vi "Length_2.vi"() -> ()   [LabVIEW 2020]
uses:
  Support/Controls/Cmd_Mouse Popup.ctl
  Support/Controls/Clst_Initialize Input.ctl
  Support/Controls/Clst_Result inspec.ctl
  Support/Controls/Cmd_Var Data IO.ctl
  Variables/Global_Cal Info.vi
panel:
  in  "불리언 2":bool=TRUE caption="평행도"
  in  "불리언 1":bool=TRUE caption="평면도"
  in  "Measured 3":string[][](table) caption="평행도"
  out "STD set":string[][](table) caption="○ 기준기 조합 (값)"
  in  "Measured 2":string[][](table) caption="평면도"
  in  "표시방식":string(combo)
  out "단위":string
  out "최대범위":string
  in  "Spec 변경":bool
  in  "Random":bool
  out "Resolution":string[][](table) caption="평면도"
  out "Spec":string[][](table) caption="평행도"
  out "제목":string
  out "에러 출력":errorcluster
  out "Condition":string[][](table) caption="2. 직선성 시험"
  in  "최소눈금":string(combo)
  in  "Measured":string[][](table) caption="평면도"
  out "Load?":bool
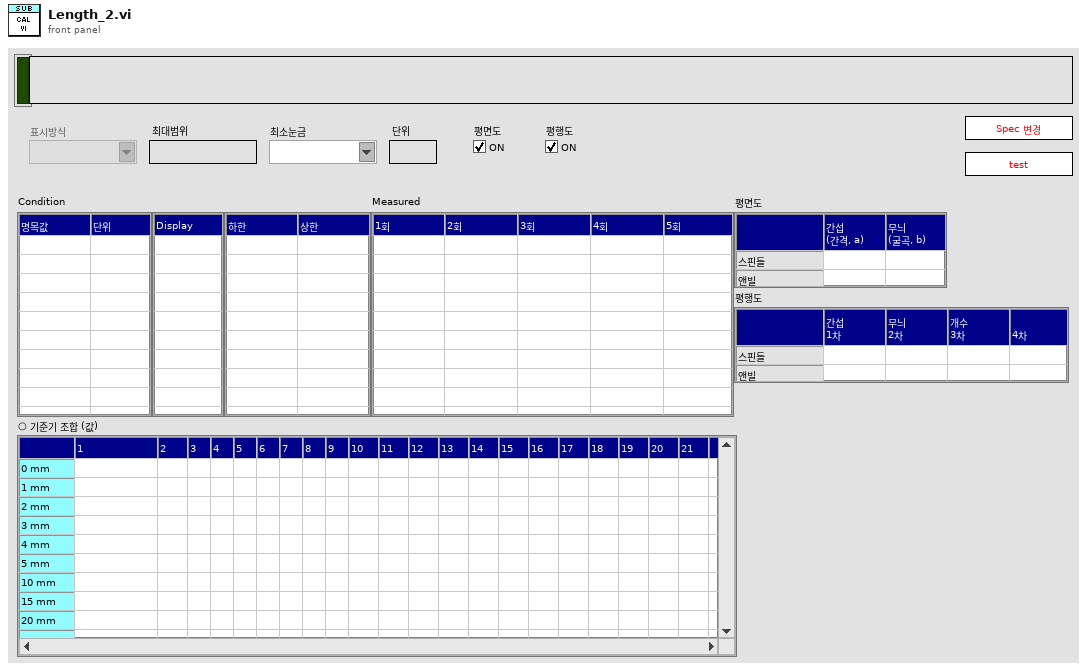
[diagram p1: front panel]
types:
  T1 = typedef "Cmd_Mouse Popup.ctl" = enum16{"활성화", "메뉴선택"}
  T2 = cluster{"Shift":bool, "Ctrl":bool, "Alt":bool, "Cmd":bool, "Opt":bool}
  T3 = typedef "Clst_Initialize Input.ctl" = cluster{"Initialize 1":cluster{"Condition":refnum<vi>[], "Spec":refnum<vi>[], "Measured":refnum<vi>[], "Resolution":refnum<vi>[], "Func_ext":string, "제목":refnum<vi>, "Measured_ADJ":refnum<vi>[]}, "Initialize 2":cluster{"문자열":refnum<vi>[], "콤보박스":refnum<vi>[], "링":refnum<vi>[], "열거형":refnum<vi>[], "테이블":refnum<vi>[], "여러열":refnum<vi>[], "디지털(DBL)":refnum<vi>[], "3D string":refnum<vi>[], "ctrl":refnum<vi>[], "boolean":refnum<vi>[]}}
  T4 = typedef "Clst_Result inspec.ctl" = cluster{"분해능":string, "문자열 1":string, "문자열 2":string, "숫자형 1":i32, "숫자형 2":i32, "숫자형 3":dbl, "문자배열 1D":string[], "문자배열 2D":string[][], "문자배열 3D":string[][][], "문자배열 4D":string[][][][], "불리언 1D":bool[]}
  T5 = typedef "Cmd_Var Data IO.ctl" = enum16{"Condition", "Condition Default", "Condition_Temp", "Resolution", "Resolution Default", "Resolution Old", "Spec", "Spec Default", "Spec Old", "Spec Temp", "Result", "Result2", "Result3", "Result_Temp", "Result_ADJ", "Result_ADJ2", "STD1", "STD2", "STD3", "STD4", "STD5", "STD Temp", "CMC", "CMC Default"}
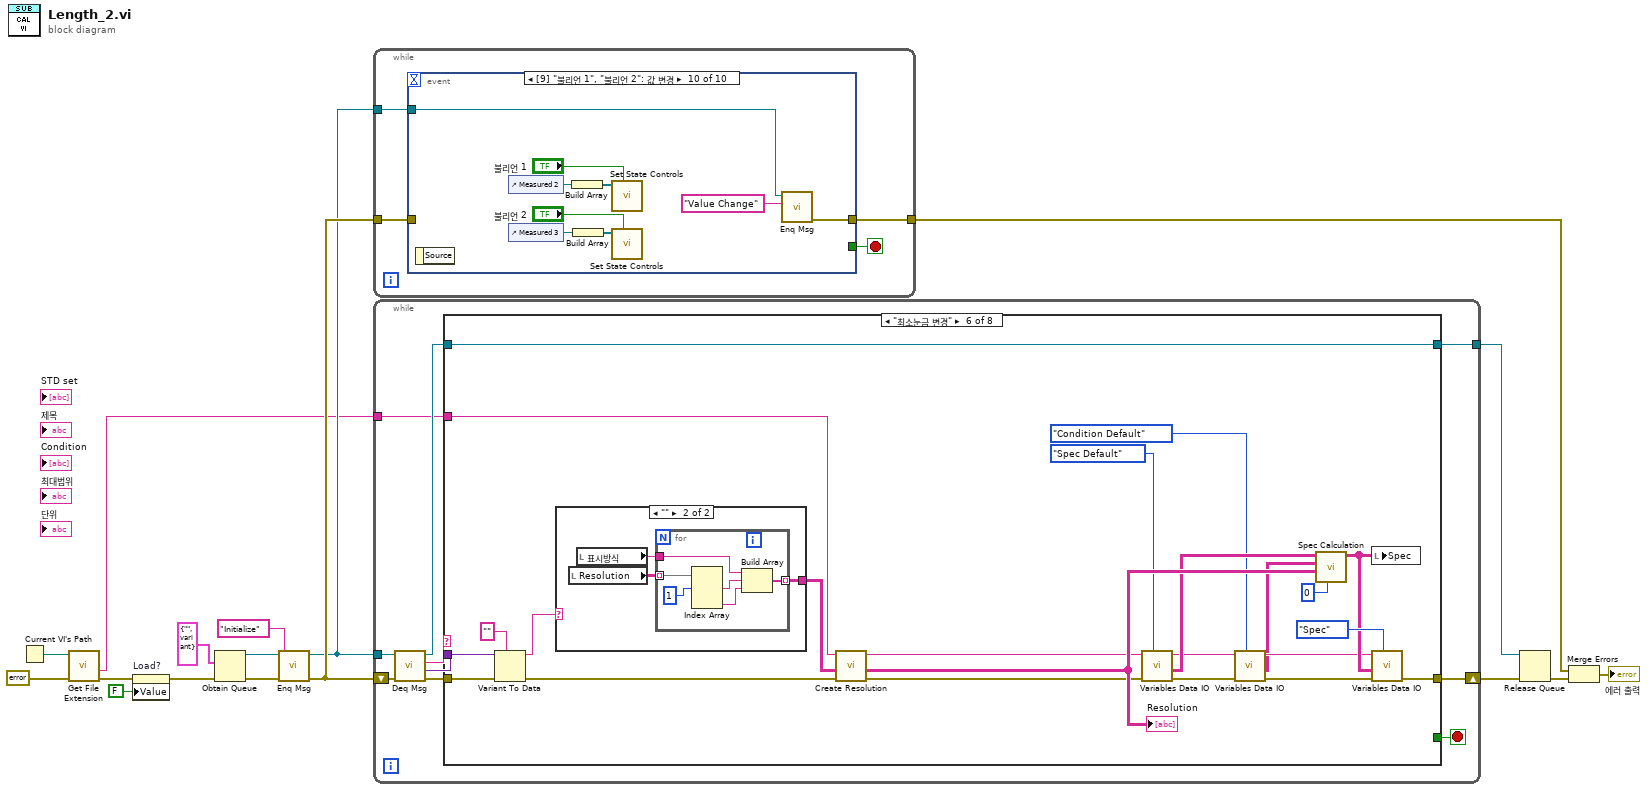
[diagram p0: block diagram]
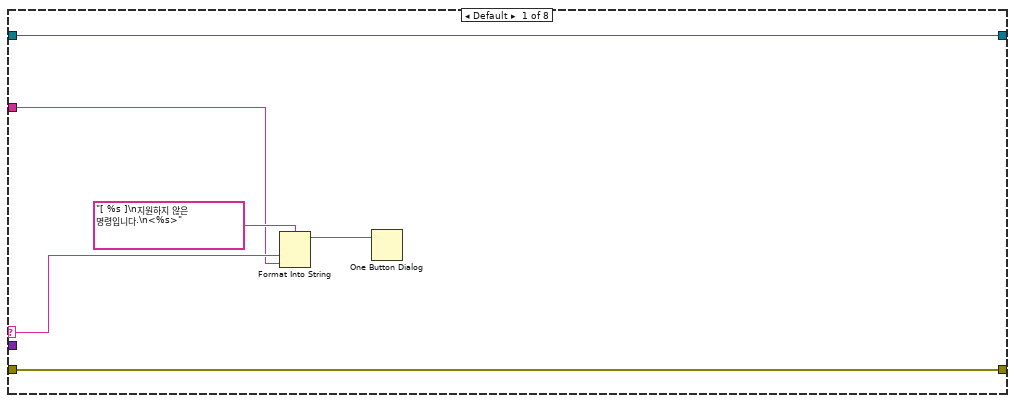
[diagram p2: hidden frame]
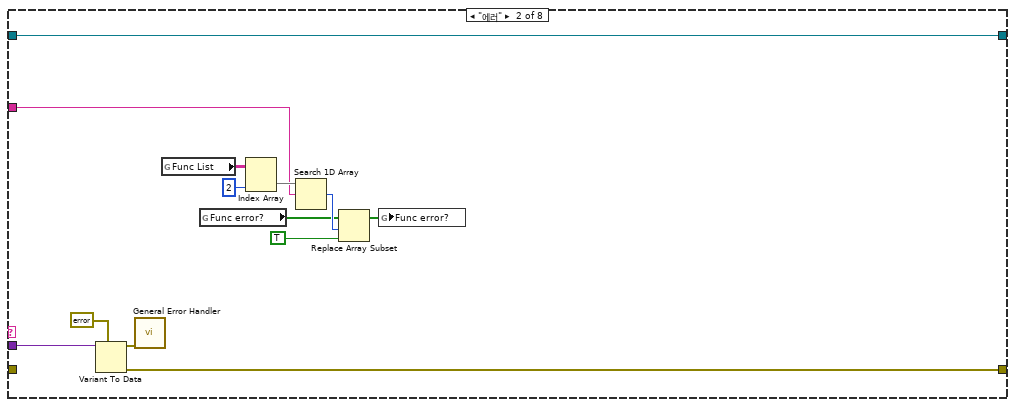
[diagram p3: hidden frame]
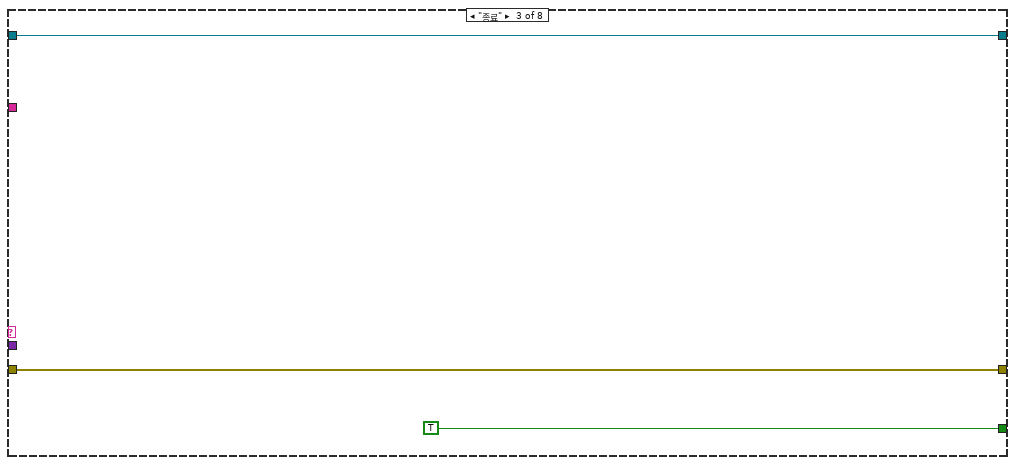
[diagram p4: hidden frame]
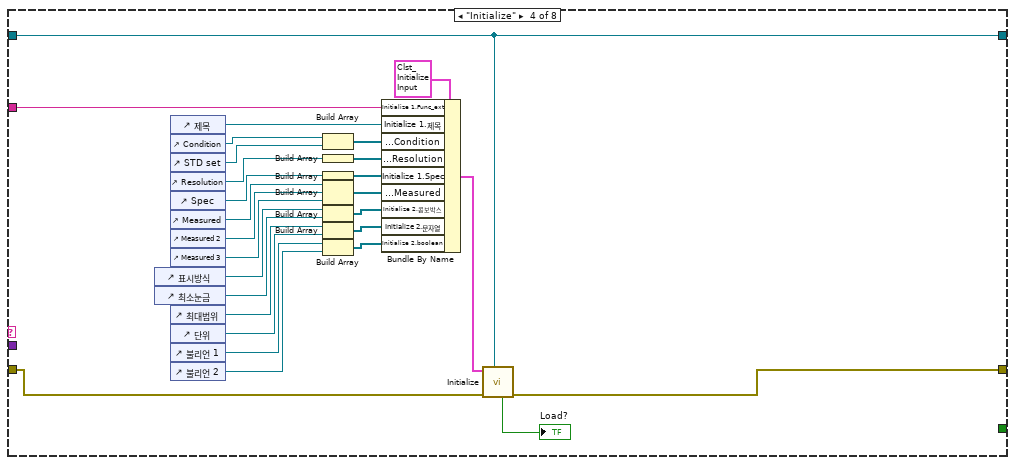
[diagram p5: hidden frame]
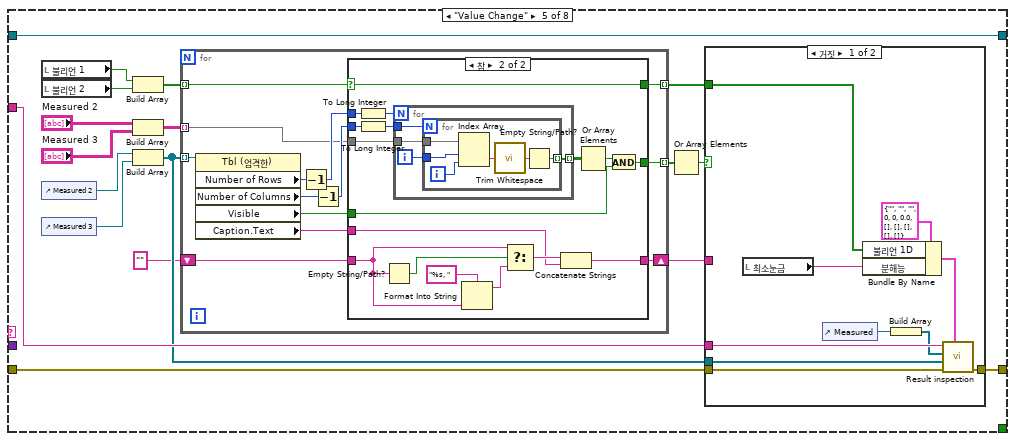
[diagram p6: hidden frame]
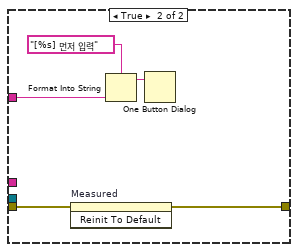
[diagram p8: hidden frame]
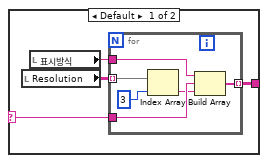
[diagram p9: hidden frame]
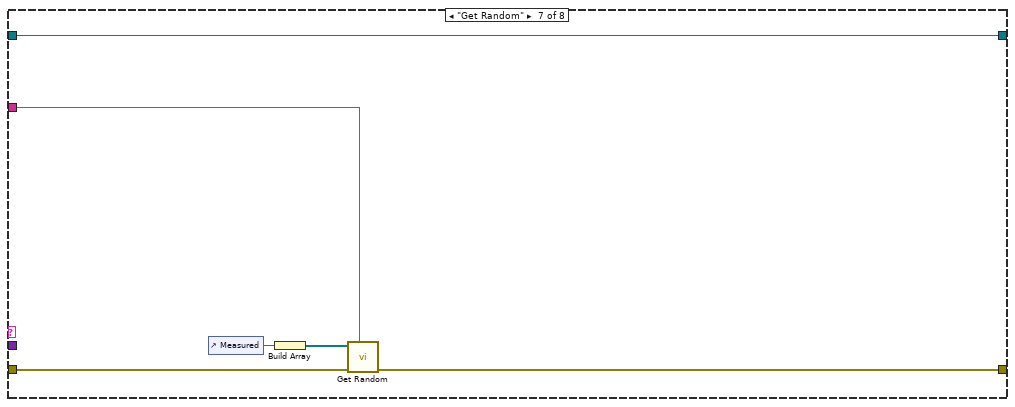
[diagram p10: hidden frame]
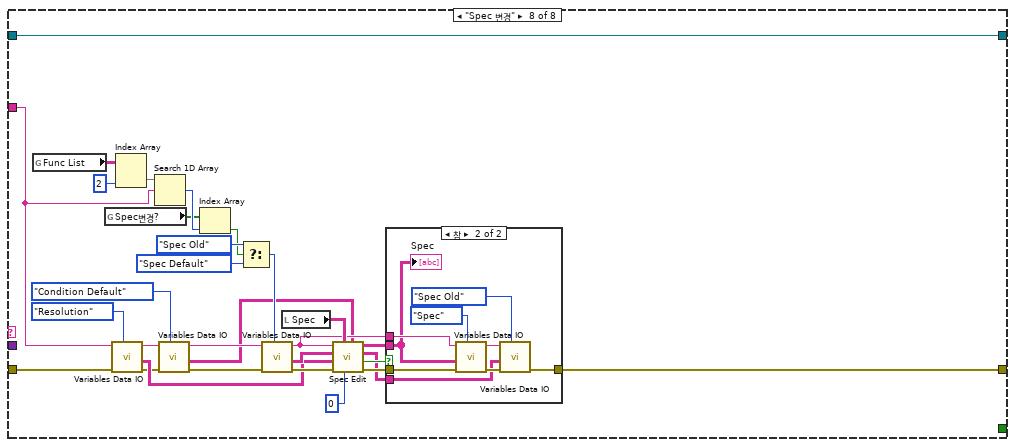
[diagram p11: hidden frame]
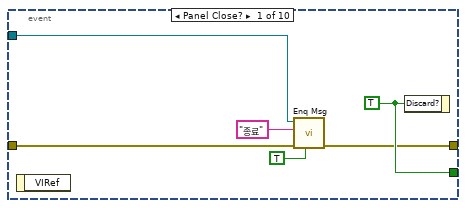
[diagram p13: hidden frame]
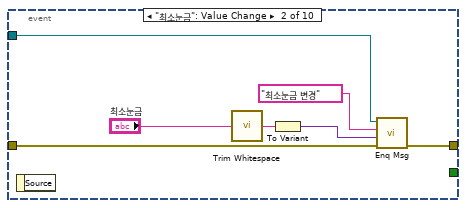
[diagram p14: hidden frame]
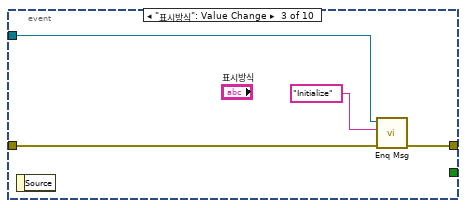
[diagram p15: hidden frame]
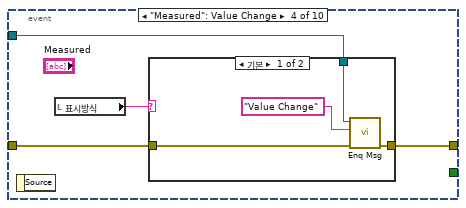
[diagram p16: hidden frame]
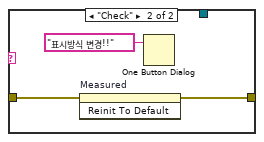
[diagram p17: hidden frame]
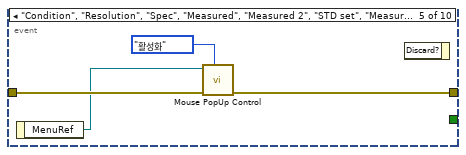
[diagram p18: hidden frame]
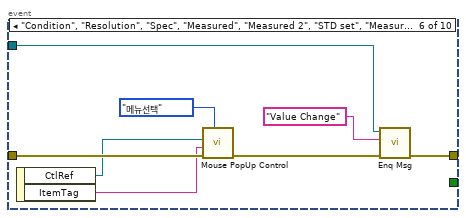
[diagram p19: hidden frame]
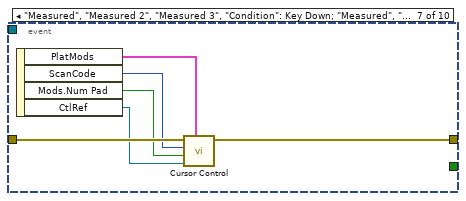
[diagram p20: hidden frame]
diagram:
  n1 = Current VI's Path() -> (path=w5:path)
  n2 = call <vilib>:"Get File Extension.vi"("error in (no error)"=errorcluster {"status"=FALSE, "code"=0, "source"=""} ("에러 상수"), "file"=w5) -> ("error out"=w3:errorcluster, "filename without extension"=w4:string)  [unwired: 5 in, 3 out]
  n3 = property on="Load?" class="Bool (엄격한)"(error in=w3, "Value"=FALSE ("Load?")) -> (error out=w2:errorcluster)  [unwired: 1 in, 1 out]
  n4 = Obtain Queue(element data type=cluster{"메세지":string, "값":variant} {"메세지"="", "값"=variant} ("Message Cluster"), error in (no error)=w2) -> (queue out=w14:refnum<queue>, error out=w16:errorcluster)  [unwired: 3 in, 1 out]
  n5 = call "Enq Msg.vi"("에러 입력(에러 없음)"=w16, "메세지"="Initialize", "큐 입력"=w14) -> ("에러 출력"=w15:errorcluster, "큐 출력"=w12:refnum<queue>)  [unwired: 7 in]
  n6 = while {
    tunnel: w15 -> [w19]
    tunnel: w12 -> [w20]
    tunnel: [w18] -> w9
    stop <- w21 stop-if-true
    n7 = event shown="[9] \"불리언 1\", \"불리언 2\": 값 변경" {
      selector: _ -> [_ _ _ _ _ _ _ _ _ _]
      dyn-events: _ -> [_ _ _ _ _ _ _ _ _ _]
      timeout: _ -> [_ _ _ _ _ _ _ _ _ _]
      tunnel: [w27 _ _ _ _ _ _ _ _ _] -> w21
      tunnel: w20 -> [w25 w33 w37 w42 _ w54 _ w72 w76 w79]
      tunnel: w19 -> [w26 w34 w38 w40 w53 w61 w67 w73 w77 _]
      tunnel: [w23 w32 w36 w41 w52 w55 w66 w68 w75 w80] -> w18
      event Panel Close? {
        w27 = TRUE ("버림?")
        n8 = event-data() -> ()  [unwired: 1 in, 1 out]
        n9 = call "Enq Msg.vi"("우선순위 메시지?"=TRUE, "에러 입력(에러 없음)"=w26, "메세지"="종료", "큐 입력"=w25) -> ("에러 출력"=w23:errorcluster)  [unwired: 6 in, 1 out]
        n10 = event-data("Discard?"=w27) -> ()  [unwired: 1 in, 1 out]
      }
      event "최소눈금": Value Change {
        n11 = event-data() -> ()  [unwired: 1 in, 1 out]
        n12 = call <vilib>:"Trim Whitespace.vi"("string"="최소눈금") -> ("trimmed string"=w30:string)  [unwired: 1 in]
        n13 = To Variant(anything=w30) -> (Variant=w28:variant)
        n14 = call "Enq Msg.vi"("에러 입력(에러 없음)"=w34, "값"=w28, "메세지"="최소눈금 변경", "큐 입력"=w33) -> ("에러 출력"=w32:errorcluster)  [unwired: 6 in, 1 out]
      }
      event "표시방식": Value Change {
        n15 = event-data() -> ()  [unwired: 1 in, 1 out]
        n16 = call "Enq Msg.vi"("에러 입력(에러 없음)"=w38, "메세지"="Initialize", "큐 입력"=w37) -> ("에러 출력"=w36:errorcluster)  [unwired: 7 in, 1 out]
      }
      event "Measured": Value Change {
        n17 = event-data() -> ()  [unwired: 1 in, 1 out]
        n18 = local read "표시방식"() -> (w39:string)
        n19 = case shown="기본" w39 {
          tunnel: w42 -> [w46 _]
          tunnel: [w45 w47] -> w41
          tunnel: w40 -> [w44 w48]
          frame Default {
            n20 = call "Enq Msg.vi"("에러 입력(에러 없음)"=w44, "메세지"="Value Change", "큐 입력"=w46) -> ("에러 출력"=w45:errorcluster)  [unwired: 7 in, 1 out]
          }
          frame "Check" {
            n21 = invoke on="Measured" class="Tbl (엄격한)" method="Reinit To Default"(error in=w48) -> (error out=w47:errorcluster)  [unwired: 2 in, 2 out]
            n22 = One Button Dialog(message="표시방식 변경!!" ("메시지")) -> ()  [unwired: 1 in, 1 out]
          }
        }
      }
      event "Condition", "Resolution", "Spec", "Measured", "Measured 2", "STD set", "Measured 3": Shortcut Menu Activation? {
        n23 = event-data() -> ("MenuRef"=w51:refnum<k9>)  [unwired: 1 in]
        n24 = call "Mouse PopUp Control.vi"("type"=Cmd_Mouse_Popup."활성화", "error in"=w53, "메뉴 참조"=w51) -> ("error out"=w52:errorcluster)  [unwired: 8 in]
        n25 = event-data() -> ()  [unwired: 2 in, 1 out]
      }
      event "Condition", "Resolution", "Spec", "Measured", "Measured 2", "STD set", "Measured 3": Shortcut Menu Selection (User) {
        n26 = event-data() -> ("CtlRef"=w59:refnum<vi>, "ItemTag"=w58:string)  [unwired: 1 in]
        n27 = call "Mouse PopUp Control.vi"("type"=Cmd_Mouse_Popup."메뉴선택", "error in"=w61, "아이템 태그"=w58, "Tbl 참조 번호"=w59) -> ("error out"=w56:errorcluster)  [unwired: 7 in]
        n28 = call "Enq Msg.vi"("에러 입력(에러 없음)"=w56, "메세지"="Value Change", "큐 입력"=w54) -> ("에러 출력"=w55:errorcluster)  [unwired: 7 in, 1 out]
      }
      event "Measured", "Measured 2", "Measured 3", "Condition": Key Down; "Measured", "Measured 2", "Measured 3", "Condition": Key Repeat {
        n29 = event-data() -> ("PlatMods"=w62:T2, "ScanCode"=w65:i16, "Mods.Num Pad"=w64:bool, "CtlRef"=w63:refnum<vi>)  [unwired: 1 in]
        n30 = call "Cursor Control.vi"("플랫폼 조합키"=w62, "참조"=w63, "Num Pad"=w64, "ScanCode"=w65, "error in"=w67) -> ("error out"=w66:errorcluster)  [unwired: 5 in, 1 out]
      }
      event "Random": Value Change {
        n31 = event-data() -> ()  [unwired: 1 in, 1 out]
        n32 = call "Enq Msg.vi"("에러 입력(에러 없음)"=w73, "메세지"="Get Random", "큐 입력"=w72) -> ("에러 출력"=w71:errorcluster, "큐 출력"=w70:refnum<queue>)  [unwired: 7 in]
        n33 = call "Enq Msg.vi"("에러 입력(에러 없음)"=w71, "메세지"="Value Change", "큐 입력"=w70) -> ("에러 출력"=w68:errorcluster)  [unwired: 7 in, 1 out]
      }
      event "Spec 변경": Value Change {
        n34 = event-data() -> ()  [unwired: 1 in, 1 out]
        n35 = call "Enq Msg.vi"("에러 입력(에러 없음)"=w77, "메세지"="Spec 변경", "큐 입력"=w76) -> ("에러 출력"=w75:errorcluster)  [unwired: 7 in, 1 out]
      }
      event "불리언 1", "불리언 2": Value Change {
        n36 = event-data() -> ()  [unwired: 1 in, 1 out]
        n37 = control-ref of="Measured 2"() -> (w87:refnum<vi>)
        n38 = control-ref of="Measured 3"() -> (w83:refnum<vi>)
        n39 = Build Array(w87) -> (w86:refnum<vi>[])
        n40 = Build Array(w83) -> (w84:refnum<vi>[])
        n41 = call "Set State Controls.vi"("활성화 (F)"="불리언 1", "컨트롤 참조 배열 in"=w86) -> ()  [unwired: 8 in, 2 out]
        n42 = call "Set State Controls.vi"("활성화 (F)"="불리언 2", "컨트롤 참조 배열 in"=w84) -> ()  [unwired: 8 in, 2 out]
        n43 = call "Enq Msg.vi"("메세지"="Value Change", "큐 입력"=w79) -> ("에러 출력"=w80:errorcluster)  [unwired: 8 in, 1 out]
      }
    }
  }
  n44 = while {
    shift-right: [w97] -> w11
    shift-left: w15 -> [w96]
    tunnel: w12 -> [w94]
    tunnel: [w89] -> w10
    tunnel: w4 -> [w88]
    stop <- w90 stop-if-true
    n45 = call "Deq Msg.vi"("에러 입력(에러 없음)"=w96, "큐 입력"=w94) -> ("에러 출력"=w95:errorcluster, "값"=w91:variant, "메세지"=w93:string, "큐 출력"=w92:refnum<queue>)  [unwired: 6 in]
    n46 = case shown="\"최소눈금 변경\"" w93 {
      selector: w93 -> [w99 _ _ _ _ _ _ _]
      tunnel: w95 -> [w103 _ w119 w147 w151 w243 w265 w292]
      tunnel: [w103 w113 w119 w137 w164 w236 w266 w295] -> w97
      tunnel: w92 -> [w102 w112 w117 w131 w165 w244 w269 w299]
      tunnel: w91 -> [_ w114 _ _ _ w242 _ _]
      tunnel: [_ _ TRUE ("버림?") _ _ _ _ _] -> w90
      tunnel: [w102 w112 w117 w131 w165 w244 w269 w299] -> w89
      tunnel: w88 -> [w98 w104 _ w132 w163 w240 w264 w277]
      frame Default {
        n47 = Format Into String(format string="[ %s ]\n지원하지 않은 명령입니다.\n<%s>" ("메시지"), w99, w98) -> (resulting string=w100:string)  [unwired: 2 in, 1 out]
        n48 = One Button Dialog(message=w100) -> ()  [unwired: 1 in, 1 out]
      }
      frame "에러" {
        n49 = Variant To Data(type=errorcluster {"status"=FALSE, "code"=0, "source"=""} ("에러 출력"), Variant=w114) -> (data=w116:errorcluster, error out=w113:errorcluster)  [unwired: 1 in]
        n50 = call <vilib>:"General Error Handler.vi"("error in (no error)"=w116) -> ()  [unwired: 10 in, 5 out]
        n51 = global read "Global_Cal Info.vi" "Func List"() -> (w106:string[][])
        n52 = global read "Global_Cal Info.vi" "Func error?"() -> (w109:bool[])
        n53 = Index Array(array=w106, index (col)=2 ("비활성화된 인덱스 (열)")) -> (element=w107:string[])  [unwired: 1 in]
        n54 = Search 1D Array(1D array=w107, element=w104) -> (index of element=w110:i32)  [unwired: 1 in]
        n55 = Replace Array Subset(array=w109, new element=TRUE ("새 원소/부분배열"), index=w110) -> (w111:bool[])
        n56 = global write "Global_Cal Info.vi" "Func error?"(w111) -> ()
      }
      frame "종료" {
      }
      frame "Initialize" {
        n57 = control-ref of="표시방식"() -> (w130:refnum<vi>)
        n58 = control-ref of="최소눈금"() -> (w140:refnum<vi>)
        n59 = control-ref of="제목"() -> (w138:refnum<vi>)
        n60 = control-ref of="Condition"() -> (w144:refnum<vi>)
        n61 = control-ref of="STD set"() -> (w125:refnum<vi>)
        n62 = control-ref of="Resolution"() -> (w133:refnum<vi>)
        n63 = control-ref of="Spec"() -> (w136:refnum<vi>)
        n64 = control-ref of="Measured"() -> (w141:refnum<vi>)
        n65 = control-ref of="Measured 2"() -> (w126:refnum<vi>)
        n66 = control-ref of="Measured 3"() -> (w124:refnum<vi>)
        n67 = control-ref of="최대범위"() -> (w127:refnum<vi>)
        n68 = control-ref of="단위"() -> (w129:refnum<vi>)
        n69 = control-ref of="불리언 1"() -> (w123:refnum<vi>)
        n70 = control-ref of="불리언 2"() -> (w122:refnum<vi>)
        n71 = Build Array(w144, w125) -> (w143:refnum<vi>[])
        n72 = Build Array(w133) -> (w134:refnum<vi>[])
        n73 = Build Array(w136) -> (w135:refnum<vi>[])
        n74 = Build Array(w141, w126, w124) -> (w142:refnum<vi>[])
        n75 = Build Array(w130, w140) -> (w139:refnum<vi>[])
        n76 = Build Array(w127, w129) -> (w128:refnum<vi>[])
        n77 = Build Array(w123, w122) -> (w121:refnum<vi>[])
        n78 = Bundle By Name(cluster=T3 {"Initialize 1"={"Condition"=[], "Spec"=[], "Measured"=[], "Resolution"=[], "Func_ext"="", "제목"=refnum, "Measured_ADJ"=[]}, "Initialize 2"={"문자열"=[], "콤보박스"=[], "링"=[], "열거형"=[], "테이블"=[], "여러열"=[], "디지털(DBL)"=[], "3D string"=[], "ctrl"=[], "boolean"=[]}} ("입력 클러스터"), "Initialize 1.Func_ext"=w132, "Initialize 1.제목"=w138, "Initialize 1.Condition"=w143, "Initialize 1.Resolution"=w134, "Initialize 1.Spec"=w135, "Initialize 1.Measured"=w142, "Initialize 2.콤보박스"=w139, "Initialize 2.문자열"=w128, "Initialize 2.boolean"=w121) -> (w145:T3)
        n79 = call "Initialize.vi"("큐 입력"=w131, "error in"=w147, "입력 클러스터"=w145) -> ("error out"=w137:errorcluster, "Load?"=→"Load?":bool)  [unwired: 5 in, 2 out]
      }
      frame "Value Change" {
        n80 = local read "불리언 1"() -> (w156:bool)
        n81 = local read "불리언 2"() -> (w157:bool)
        n82 = control-ref of="Measured 2"() -> (w154:refnum<vi>)
        n83 = control-ref of="Measured 3"() -> (w160:refnum<vi>)
        n84 = Build Array(w156, w157) -> (w158:bool[])
        n85 = Build Array("Measured 2", "Measured 3") -> (w155:string[][][])
        n86 = Build Array(w154, w160) -> (w152:refnum<vi>[])
        n87 = for {
          tunnel: w152 -> [w178] mode=indexing
          tunnel: w155 -> [w173] mode=indexing
          tunnel: w158 -> [w170] mode=indexing
          tunnel: [w169] -> w159 mode=indexing
          shift-right: [w167] -> w149
          shift-left: "" ("Caption.Text") -> [w168]
          tunnel: [w166] -> w148 mode=indexing
          n88 = property on="프로퍼티 노드" class="Tbl (엄격한)"(reference=w178) -> ("Number of Rows"=w177:u32, "Number of Columns"=w176:u32, "Visible"=w172:bool, "Caption.Text"=w171:string)  [unwired: 1 in, 2 out]
          n89 = Decrement(x=w177) -> (x-1=w175:u32)
          n90 = Decrement(x=w176) -> (x-1=w174:u32)
          n91 = case shown="참" w170 {
            selector: w170 -> [_ w180]
            tunnel: w173 -> [_ w192]
            tunnel: w175 -> [_ w196]
            tunnel: w172 -> [_ w189]
            tunnel: w174 -> [_ w195]
            tunnel: [_ w188] -> w169
            tunnel: w171 -> [_ w181]
            tunnel: w168 -> [w179 w183]
            tunnel: [w179 w182] -> w167
            tunnel: [_ w180] -> w166
            frame False {
            }
            frame True {
              n92 = To Long Integer(number=w196) -> (32bit integer=w194:i32)
              n93 = To Long Integer(number=w195) -> (32bit integer=w193:i32)
              n94 = Empty String/Path?(string/path=w183) -> (empty?=w187:bool)
              n95 = for {
                N: w194 -> [_]
                tunnel: w192 -> [w199]
                tunnel: w193 -> [w200]
                tunnel: [w198] -> w191 mode=indexing
                i -> [w197]
                n96 = for {
                  N: w200 -> [_]
                  tunnel: w199 -> [w204]
                  tunnel: [w205] -> w198 mode=indexing
                  tunnel: w197 -> [w202]
                  i -> [w201]
                  n97 = Index Array(array=w204, index (row)=w202, index (col)=w201) -> (element=w203:string)
                  n98 = call <vilib>:"Trim Whitespace.vi"("string"=w203) -> ("trimmed string"=w206:string)  [unwired: 1 in]
                  n99 = Empty String/Path?(string/path=w206) -> (empty?=w205:bool)
                }
              }
              n100 = Format Into String(format string="%s, " ("포맷 문자열"), w183) -> (resulting string=w185:string)  [unwired: 2 in, 1 out]
              n101 = Select(t=w183, s=w187, f=w185) -> (s? t:f=w184:string)
              n102 = Concatenate Strings(w184, w181) -> (w182:string)
              n103 = Or Array Elements(Boolean array=w191) -> (logical OR=w190:bool)
              n104 = And(x=w190, y=w189) -> (x .and. y?=w188:bool)
            }
          }
        }
        n105 = Or Array Elements(Boolean array=w159) -> (logical OR=w153:bool)
        n106 = case shown="거짓" w153 {
          tunnel: [w216 w219] -> w164
          tunnel: w163 -> [w215 _]
          tunnel: w152 -> [w209 _]
          tunnel: w151 -> [w208 w218]
          tunnel: w149 -> [_ w217]
          tunnel: w148 -> [w207 _]
          frame False {
            n107 = local read "최소눈금"() -> (w211:string)
            n108 = control-ref of="Measured"() -> (w214:refnum<vi>)
            n109 = Bundle By Name(cluster=T4 {"분해능"="", "문자열 1"="", "문자열 2"="", "숫자형 1"=0, "숫자형 2"=0, "숫자형 3"=0.0, "문자배열 1D"=[], "문자배열 2D"=[], "문자배열 3D"=[], "문자배열 4D"=[], "불리언 1D"=[]} ("입력 클러스터"), "불리언 1D"=w207, "분해능"=w211) -> (w210:T4)
            n110 = Build Array(w214) -> (w213:refnum<vi>[])
            n111 = call "Result inspection.vi"("입력 클러스터"=w210, "error in"=w208, "Ref. Data (excluded)"=w209, "Ref. Data (Inspection)"=w213, "Func ext"=w215) -> ("error out"=w216:errorcluster)  [unwired: 3 in, 3 out]
          }
          frame True {
            n112 = invoke on="Measured" class="Tbl (엄격한)" method="Reinit To Default"(error in=w218) -> (error out=w219:errorcluster)  [unwired: 2 in, 2 out]
            n113 = Format Into String(format string="[%s] 먼저 입력" ("포맷 문자열"), w217) -> (resulting string=w220:string)  [unwired: 2 in, 1 out]
            n114 = One Button Dialog(message=w220) -> ()  [unwired: 1 in, 1 out]
          }
        }
      }
      frame "최소눈금 변경" {
        n115 = Variant To Data(error in=w243, type="", Variant=w242) -> (data=w229:string, error out=w231:errorcluster)
        n116 = case shown="\"\"" w229 {
          selector: w229 -> [w245 _]
          tunnel: [w248 w257] -> w230
          frame Default {
            n117 = local read "Resolution"() -> (w247:string[][])
            n118 = local read "표시방식"() -> (w246:string)
            n119 = for {
              tunnel: w247 -> [w254] mode=indexing
              tunnel: w245 -> [w253]
              tunnel: [w251] -> w248 mode=indexing
              tunnel: w246 -> [w250]
              n120 = Index Array(array=w254, index=3 ("인덱스")) -> (element=w252:string)
              n121 = Build Array(w250, w253, w252) -> (w251:string[])
            }
          }
          frame "" {
            n122 = local read "Resolution"() -> (w256:string[][])
            n123 = local read "표시방식"() -> (w255:string)
            n124 = for {
              tunnel: w256 -> [w263] mode=indexing
              tunnel: [w262] -> w257 mode=indexing
              tunnel: w255 -> [w261]
              n125 = Index Array(array=w263, index #1=1 ("인덱스")) -> (element #1=w259:string, element #3=w258:string)  [unwired: 2 in, 1 out]
              n126 = Build Array(w261, w259, w258) -> (w262:string[])
            }
          }
        }
        n127 = call "Create Resolution.vi"("에러 입력(에러 없음)"=w231, "Resolution"=w230, "Func_ext"=w240) -> ("에러 출력"=w234:errorcluster, "Resolution Out"=w237:string[][], "Func_ext 출력"=w233:string)  [unwired: 6 in]
        "Resolution" <- w237
        n128 = call "Variables Data IO.vi"("Select"=Cmd_Var_Data_IO."Spec Default", "error in"=w234, "Func_ext"=w233) -> ("error out"=w225:errorcluster, "Data Out"=w232:string[][], "Func_ext Out"=w226:string)  [unwired: 6 in]
        n129 = call "Variables Data IO.vi"("Select"=Cmd_Var_Data_IO."Condition Default", "error in"=w225, "Func_ext"=w226) -> ("error out"=w223:errorcluster, "Data Out"=w222:string[][], "Func_ext Out"=w224:string)  [unwired: 6 in]
        n130 = call "Spec Calculation.vi"("기준값 열번호"=0 ("열번호(기준값)"), "Resolution"=w237, "Condition in"=w222, "Spec Default"=w232) -> ("Spec out"=w228:string[][])  [unwired: 6 in, 1 out]
        n131 = local write "Spec"(w228) -> ()
        n132 = call "Variables Data IO.vi"("Select"=Cmd_Var_Data_IO."Spec", "error in"=w223, "Data In"=w228, "Func_ext"=w224) -> ("error out"=w236:errorcluster)  [unwired: 5 in, 2 out]
      }
      frame "Get Random" {
        n133 = control-ref of="Measured"() -> (w268:refnum<vi>)
        n134 = Build Array(w268) -> (w267:refnum<vi>[])
        n135 = call "Get Random.vi"("Func_Ext"=w264, "에러 입력"=w265, "Meas"=w267) -> ("에러 출력"=w266:errorcluster)  [unwired: 7 in, 1 out]
      }
      frame "Spec 변경" {
        n136 = global read "Global_Cal Info.vi" "Func List"() -> (w282:string[][])
        n137 = global read "Global_Cal Info.vi" "Spec변경?"() -> (w278:bool[])
        n138 = call "Variables Data IO.vi"("Select"=Cmd_Var_Data_IO."Resolution", "error in"=w292, "Func_ext"=w277) -> ("error out"=w275:errorcluster, "Data Out"=w286:string[][], "Func_ext Out"=w273:string)  [unwired: 6 in]
        n139 = Index Array(array=w282, index (col)=2 ("비활성화된 인덱스 (열)")) -> (element=w280:string[])  [unwired: 1 in]
        n140 = Search 1D Array(1D array=w280, element=w277) -> (index of element=w279:i32)  [unwired: 1 in]
        n141 = call "Variables Data IO.vi"("Select"=Cmd_Var_Data_IO."Condition Default", "error in"=w275, "Func_ext"=w273) -> ("error out"=w274:errorcluster, "Data Out"=w270:string[][], "Func_ext Out"=w272:string)  [unwired: 6 in]
        n142 = Index Array(array=w278, index=w279) -> (element=w283:bool)
        n143 = Select(t=Cmd_Var_Data_IO."Spec Old" ("Select"), s=w283, f=Cmd_Var_Data_IO."Spec Default" ("Select")) -> (s? t:f=w276:T5)
        n144 = call "Variables Data IO.vi"("Select"=w276, "error in"=w274, "Func_ext"=w272) -> ("error out"=w294:errorcluster, "Data Out"=w287:string[][], "Func_ext Out"=w288:string)  [unwired: 6 in]
        n145 = local read "Spec"() -> (w289:string[][])
        n146 = call "Spec Edit.vi"("Condition"=w270, "열번호(기준값)"=0, "Spec Value"=w289, "에러 입력(에러 없음)"=w294, "Resolution"=w286, "Spec Default"=w287, "Func_ext"=w288) -> ("에러 출력"=w296:errorcluster, "변경?"=w297:bool, "Spec Default out"=w291:string[][], "Spec 출력"=w298:string[][])  [unwired: 1 in]
        n147 = case shown="참" w297 {
          tunnel: w298 -> [_ w306]
          tunnel: w296 -> [w300 w309]
          tunnel: [w300 w304] -> w295
          tunnel: w288 -> [_ w307]
          tunnel: w291 -> [_ w302]
          frame False {
          }
          frame True {
            n148 = call "Variables Data IO.vi"("Select"=Cmd_Var_Data_IO."Spec", "error in"=w309, "Data In"=w306, "Func_ext"=w307) -> ("error out"=w305:errorcluster, "Func_ext Out"=w303:string)  [unwired: 5 in, 1 out]
            n149 = call "Variables Data IO.vi"("Select"=Cmd_Var_Data_IO."Spec Old", "error in"=w305, "Data In"=w302, "Func_ext"=w303) -> ("error out"=w304:errorcluster)  [unwired: 5 in, 2 out]
            "Spec" <- w306
          }
        }
      }
    }
  }
  n150 = Release Queue(queue=w10, error in (no error)=w11) -> (error out=w8:errorcluster)  [unwired: 1 in, 2 out]
  n151 = Merge Errors(w9, w8) -> (→"에러 출력":errorcluster)
